vi "PH_Beamline.set BB State in GUI.vi"(0 "i ref in":refnum<vi>, 1 "Boolean GUI Ref":refnum<vi>, 2 "Picture GUI Ref":refnum<vi>, 3 "Status":T1 items=["no info", "off/false/out", "on/true/in", "Failure", "Alarm", "Status 1", "Status 2", "Status 3"], 4 "no Link?":bool, 5 "error in":errorcluster) -> (14 "i ref out":refnum<vi>, 19 "error out":errorcluster)   [LabVIEW 2014, in "PH_Beamline.lvlib"]
doc: "This VI sets the BB GUI object."
uses:
  PH_Beamline.lvlib
  PH_StatusHandler/PH_StatusHandler.Status.ctl
  PH_BL-Master/PH_BL-Master.Shutter State.ctl
  PH_Beamline.Black Box Instances.ctl
  PH_Common/Picture/PH_Picture.Alignment.ctl
  PH_Common/PH_Common.lvlib
  PH_Beamline_Common/PH_Beamline_Common.lvlib
  PH_StatusHandler/PH_StatusHandler.lvlib
  PH_BL-Master/PH_BL-Master.lvlib
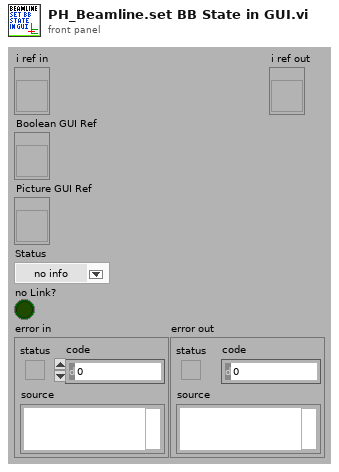
[diagram p1: front panel]
types:
  T1 = typedef "PH_StatusHandler.lvlib/PH_StatusHandler.Status.ctl" = i16
  T2 = typedef "PH_Beamline.lvlib/PH_Beamline.Black Box Instances.ctl" = string
  T3 = typedef "PH_BL-Master.lvlib/PH_BL-Master.Shutter State.ctl" = enum16{"No Link", "No Info", "In", "Out", "in between"}
  T4 = enum16{"No Link", "No Info", "In", "Out", "in between"}
  T5 = typedef "PH_Common.lvlib/PH_Picture.Alignment.ctl" = enum16{"neutral", "left", "right", "up", "down", "vertical", "horizontal", "left down to right up", "left up to right down"}
  T6 = typedef "PH_BL-Master.lvlib/PH_BL-Master.i attribute.ctl" = cluster{"Remote controlled":bool, "Boolean Condition Service Subscriber":refnum<vi>[], "Picture Condition Service Subscriber":refnum<vi>[], "R2S":cluster{"GUI Ref":refnum<vi>, "State":bool}, "Vacua":cluster{"GUI Ref":refnum<vi>, "Limit":dbl, "Curr Value":dbl, "in range":bool}[], "O2 Inspection":cluster{"GUI Ref":refnum<vi>, "Concentration":dbl, "State":T1}[], "Boolean Status Service Subscriber":cluster{"GUI Ref":refnum<vi>, "Status":T1, "no Link?":bool, "Status Subscriber Class":T7}[], "Picture Status Service Subscriber":cluster{"GUI Ref":refnum<vi>, "Status":T1, "no Link?":bool, "Status Subscriber Class":T7}[], "6P 4Q Service Subscriber":cluster{"GUI Ref":refnum<vi>, "Selector":T8, "no Link?":bool}[], "Index of latest 6P 4Q changing Instance":i32, "Index of latest Picture Status changing Instance":i32, "Index of latest Boolean Status changing Instance":i32, "Vision ID on same Node":string, "Start Phase over?":bool, "GUI Ref Delete":refnum<vi>}
  T7 = typedef "PH_BL-Master.lvlib/PH_BL-Master.Status Subscriber Class.ctl" = enum16{"unknown", "Switch", "BB", "6P Switch", "Switch GUI", "Switch and 6P State", "Force Sensor"}
  T8 = typedef "PH_4_Pos_Selector.lvlib/PH_4_Pos_Selector.Position Selector.ctl" = u16
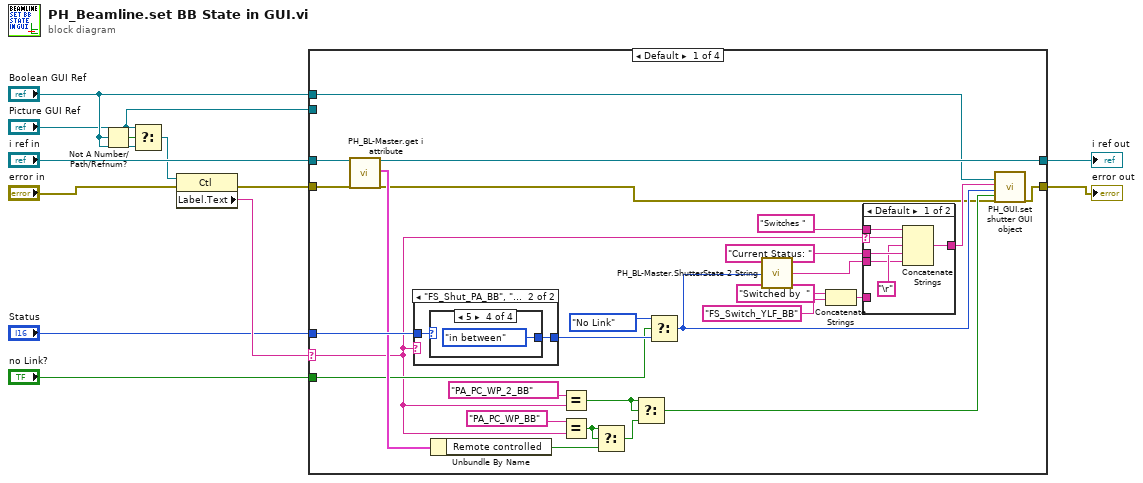
[diagram p0: block diagram]
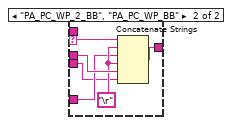
[diagram p2: hidden frame]
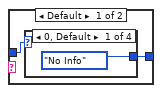
[diagram p3: hidden frame]
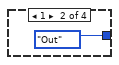
[diagram p4: hidden frame]
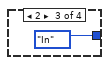
[diagram p5: hidden frame]
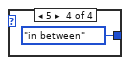
[diagram p6: hidden frame]
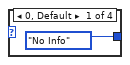
[diagram p7: hidden frame]
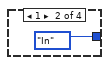
[diagram p8: hidden frame]
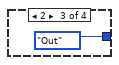
[diagram p9: hidden frame]
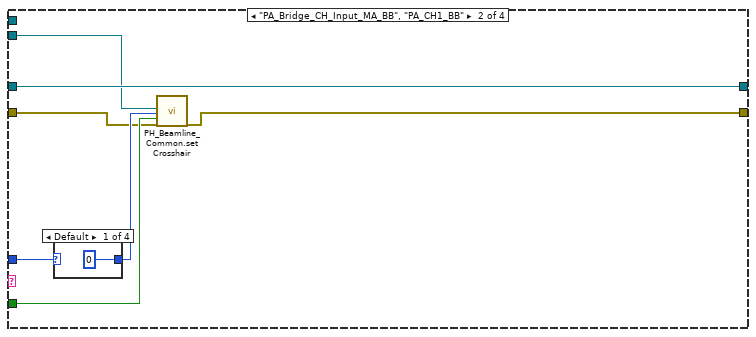
[diagram p10: hidden frame]
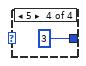
[diagram p13: hidden frame]
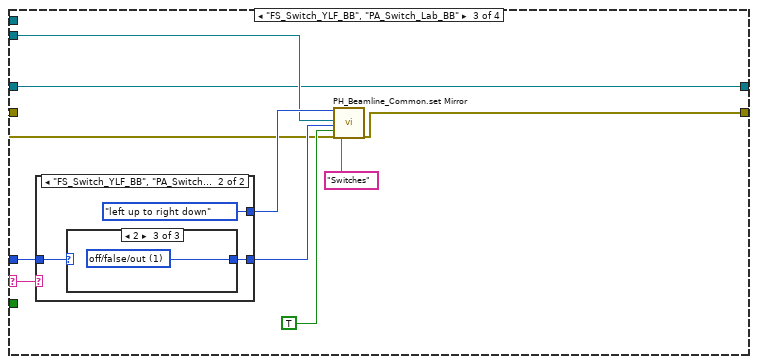
[diagram p14: hidden frame]
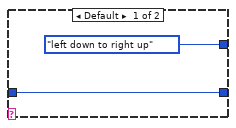
[diagram p15: hidden frame]
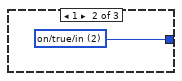
[diagram p17: hidden frame]
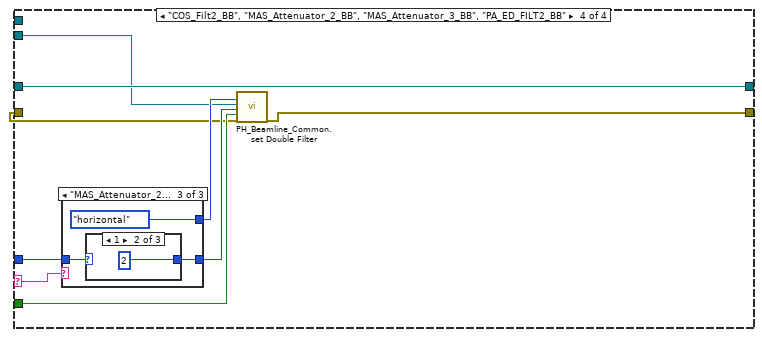
[diagram p18: hidden frame]
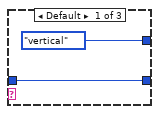
[diagram p19: hidden frame]
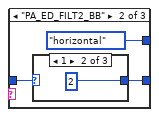
[diagram p20: hidden frame]
diagram:
  n1 = Not A Number/Path/Refnum?(number/path/refnum="Boolean GUI Ref") -> (NaN/Path/Refnum?=w8:bool)
  n2 = Select(t="Picture GUI Ref", s=w8, f="Boolean GUI Ref") -> (s? t:f=w9:refnum<vi>)
  n3 = property class="Ctl"(reference=w9, error in="error in") -> (error out=w6:errorcluster, "Label.Text"=w5:string)  [unwired: 1 out]
  n4 = case "Empty name, Double Filter, crosshairs and other BBs" shown="Default" w5 {
    selector: w5 -> [w16 _ w82 w97]
    tunnel: "Status" -> [w39 w70 w81 w99]
    tunnel: [w38 w69 w84 w101] -> w12
    tunnel: [w37 w65 w75 w94] -> w11
    tunnel: "i ref in" -> [w35 w65 w75 w94]
    tunnel: w6 -> [w34 w66 w76 w95]
    tunnel: "no Link?" -> [w25 w68 _ w100]
    tunnel: "Boolean GUI Ref" -> [w14 _ _ _]
    tunnel: "Picture GUI Ref" -> [_ w64 w77 w93]
    frame Default {
      n5 = call "PH_BL-Master.get i attribute.vi"("i ref in"=w35, "error in (no error)"=w34) -> ("i ref out"=w37:refnum<vi>, "i attribute"=w36:T6, "error out"=w15:errorcluster)  [unwired: 15 in]
      n6 = case shown="\"FS_Shut_PA_BB\", \"MAS_Attenuator_1_BB\", \"MA_Diffusor_Inject_In_BB\", \"NS_Shut_PA_BB\", \"PA_ED_FILT1_BB\", \"PA_Exit_Shut_BB\", \"PA_LL_CH_Input_BB\", \"PA_Shut_Input_BB\"" w16 {
        tunnel: [w53 w59] -> w31
        tunnel: w39 -> [w52 w58]
        frame Default {
          n7 = case shown="0, Default" w52 {
            tunnel: [T4."No Info" ("Shutter State") T4."Out" ("Shutter State") T4."In" ("Shutter State") T4."in between" ("Shutter State")] -> w53
            frame 0, Default {
            }
            frame 1 {
            }
            frame 2 {
            }
            frame 5 {
            }
          }
        }
        frame "FS_Shut_PA_BB", "MAS_Attenuator_1_BB", "MA_Diffusor_Inject_In_BB", "NS_Shut_PA_BB", "PA_ED_FILT1_BB", "PA_Exit_Shut_BB", "PA_LL_CH_Input_BB", "PA_Shut_Input_BB" {
          n8 = case shown="5" w58 {
            tunnel: [PH_BL-Master.Shutter_State."No Info" ("Shutter State") PH_BL-Master.Shutter_State."In" ("Shutter State") PH_BL-Master.Shutter_State."Out" ("Shutter State") PH_BL-Master.Shutter_State."in between" ("Shutter State")] -> w59
            frame 0, Default {
            }
            frame 1 {
            }
            frame 2 {
            }
            frame 5 {
            }
          }
        }
      }
      n9 = Unbundle By Name(w36) -> ("Remote controlled"=w13:bool)
      n10 = Equal?(x=T2 "PA_PC_WP_2_BB" ("Black Box Instances"), y=w16) -> (x = y?=w28:bool)
      n11 = Equal?(x=T2 "PA_PC_WP_BB" ("Black Box Instances 2"), y=w16) -> (x = y?=w33:bool)
      n12 = Select(t=w33, s=w33, f=w13) -> (s? t:f=w27:bool)
      n13 = Select(t=w28, s=w28, f=w27) -> (s? t:f=w26:bool)
      n14 = Select(t=PH_BL-Master.Shutter_State."No Link" ("Shutter State"), s=w25, f=w31) -> (s? t:f=w17:T3)
      n15 = call "PH_BL-Master.ShutterState 2 String.vi"("Shutter State"=w17) -> ("String"=w18:string)
      n16 = Concatenate Strings("Switched by  " ("string"), T2 "FS_Switch_YLF_BB" ("Black Box Instances")) -> (w20:string)
      n17 = case shown="Default" w16 {
        selector: w16 -> [w41 w47]
        tunnel: [w45 w51] -> w19
        tunnel: "Current Status: " ("string") -> [w44 w50]
        tunnel: w18 -> [w40 w46]
        tunnel: "Switches " ("string") -> [w42 _]
        tunnel: w20 -> [_ w48]
        frame Default {
          n18 = Concatenate Strings(w42, w41, "\r", w44, w40) -> (w45:string)
        }
        frame "PA_PC_WP_2_BB", "PA_PC_WP_BB" {
          w49 = "\r"
          n19 = Concatenate Strings(w47, w49, w48, w49, w50, w46) -> (w51:string)
        }
      }
      n20 = call "PH_GUI.set shutter GUI object.vi"("Wanted Boolean Ref"=w14, "Tip Strip"=w19, "Shutter State"=w17, "Disabled? (false)"=w26, "error in (no error)"=w15) -> ("error out"=w38:errorcluster)  [unwired: 14 in]
    }
    frame "PA_Bridge_CH_Input_MA_BB", "PA_CH1_BB" {
      n21 = case shown="Default" w70 {
        selector: w70 -> [_ w72 w73 _]
        tunnel: [i16 0 ("Cross Hair Status") w72 w73 i16 3 ("Cross Hair Status")] -> w67
        frame Default {
        }
        frame 1 {
        }
        frame 2 {
        }
        frame 5 {
        }
      }
      n22 = call "PH_Beamline_Common.set Crosshair.vi"("CtlRef"=w64, "State"=w67, "no link"=w68, "error in (no error)"=w66) -> ("error out"=w69:errorcluster)  [unwired: 15 in]
    }
    frame "FS_Switch_YLF_BB", "PA_Switch_Lab_BB" {
      n23 = case shown="\"FS_Switch_YLF_BB\", \"PA_Switch_Lab_BB\"" w82 {
        tunnel: [w86 w88] -> w80
        tunnel: w81 -> [w86 w89]
        tunnel: [PH_Picture.Alignment."left down to right up" ("Alignment (left down to right up)") PH_Picture.Alignment."left up to right down" ("Alignment (left down to right up)")] -> w79
        frame Default {
        }
        frame "FS_Switch_YLF_BB", "PA_Switch_Lab_BB" {
          n24 = case shown="2" w89 {
            selector: w89 -> [w90 _ _]
            tunnel: [w90 w91 w92] -> w88
            frame Default {
            }
            frame 1 {
              w91 = T1 2 items=["no info", "off/false/out", "on/true/in", "Failure", "Alarm", "Status 1", "Status 2", "Status 3"] ("Status (on/true/in)")
            }
            frame 2 {
              w92 = T1 1 items=["no info", "off/false/out", "on/true/in", "Failure", "Alarm", "Status 1", "Status 2", "Status 3"] ("Status (on/true/in)")
            }
          }
        }
      }
      n25 = call "PH_Beamline_Common.set Mirror.vi"("Alignment (left down to right up)"=w79, "CtlRef"=w77, "Status (on/true/in)"=w80, "GUI Instance does not exist or here?"=TRUE, "error in (no error)"=w76, "Tip Strip (N/A)"="Switches") -> ("error out"=w84:errorcluster)  [unwired: 13 in]
    }
    frame "COS_Filt2_BB", "MAS_Attenuator_2_BB", "MAS_Attenuator_3_BB", "PA_ED_FILT2_BB" {
      n26 = case shown="\"MAS_Attenuator_2_BB\", \"MAS_Attenuator_3_BB\"" w97 {
        tunnel: [w103 w105 w111] -> w98
        tunnel: [PH_Picture.Alignment."vertical" ("Alignment (vertical)") PH_Picture.Alignment."horizontal" ("Alignment (vertical)") PH_Picture.Alignment."horizontal" ("Alignment (vertical)")] -> w96
        tunnel: w99 -> [w103 w106 w112]
        frame Default {
        }
        frame "PA_ED_FILT2_BB" {
          n27 = case shown="1" w106 {
            selector: w106 -> [w107 _ _]
            tunnel: [w107 i16 2 ("State") i16 1 ("State")] -> w105
            frame Default {
            }
            frame 1 {
            }
            frame 2 {
            }
          }
        }
        frame "MAS_Attenuator_2_BB", "MAS_Attenuator_3_BB" {
          n28 = case shown="1" w112 {
            selector: w112 -> [w113 _ _]
            tunnel: [w113 i16 2 ("State") i16 1 ("State")] -> w111
            frame Default {
            }
            frame 1 {
            }
            frame 2 {
            }
          }
        }
      }
      n29 = call "PH_Beamline_Common.set Double Filter.vi"("Alignment (vertical)"=w96, "CtlRef"=w93, "State"=w98, "no link"=w100, "error in (no error)"=w95) -> ("error out"=w101:errorcluster)  [unwired: 14 in]
    }
  }
  "error out" <- w12
  "i ref out" <- w11
